vi "OxfordDC_2Channel_ITC503_LKS331_2SRS830.vi"() -> ()   [LabVIEW 2014]
uses:
  <vilib>/Utility/file.llb/Write To Spreadsheet File (DBL).vi
  Lake Shore Cryotronics 370/Lake Shore Cryotronics 370.lvlib
panel:
  out "Probe Temp":dbl format="%.3f"
  out "Cryostat Temp":dbl format="%.3f"
  in  "Tab Control":enum32{"Page 1", "Page 3"}(tab)
  in  "Start T":dbl=130.0
  in  "T Step":dbl=1.0
  in  "End T":dbl
  in  "Mid T":dbl
  in  "T Step 2":dbl=1.0
  in  "Seconds for Stability":dbl=200.0
  in  "SRS830_1\nAddress":i16
  in  "SRS830_2\nAddress":i16
  in  "Save file path":path
  in  "error in (no error)":errorcluster
  out "error out":errorcluster
  in  "Amplitude":dbl=0.75
  in  "Delay Time (s)":dbl=0.4
  in  "Frequency":dbl=0.1
  in  "Offset":dbl=3.0
  in  "Phase":dbl
  in  "Amplifier Offset":dbl=0.1 caption="Frequency"
  in  "Amplifier Gain":dbl=0.1 caption="Frequency"
  in  "Setpoint Proximity":dbl=0.01 format="%#.3g"
  in  "Required Stability":dbl=0.002 format="%#.4g"
  in  "ITC503":refnum<visa-resource-name>
  in  "LKS 370":refnum<visa-resource-name>
  out "XY Graph 3":cluster{dbl, dbl}[](graph) caption="SRS2"
  out "XY Graph 4":cluster{dbl, dbl}[](graph) caption="SRS1"
  out "XY Graph 5":cluster{dbl, dbl}[](graph) caption="LR700"
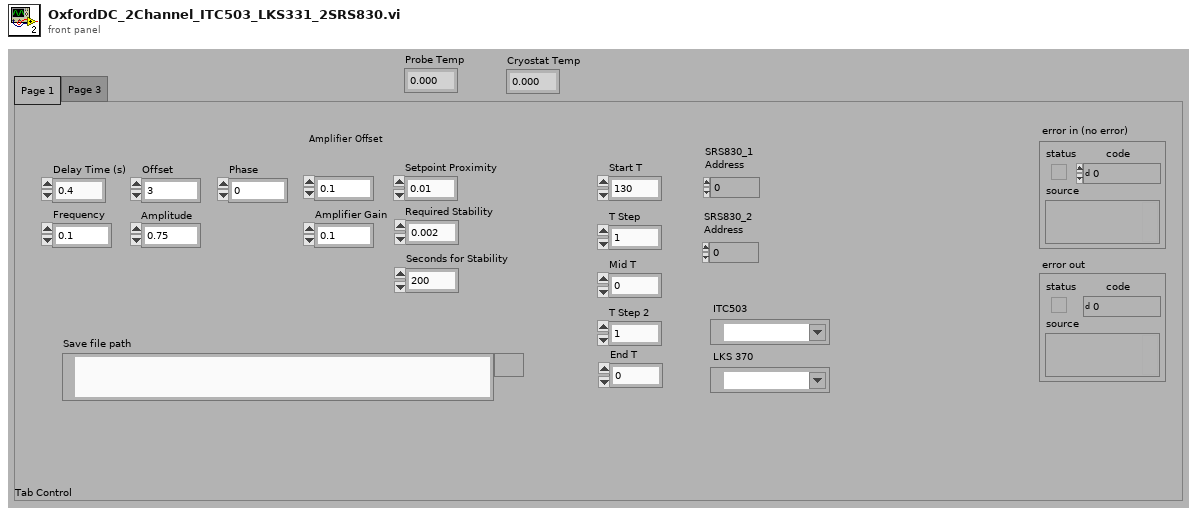
[diagram p1: front panel]
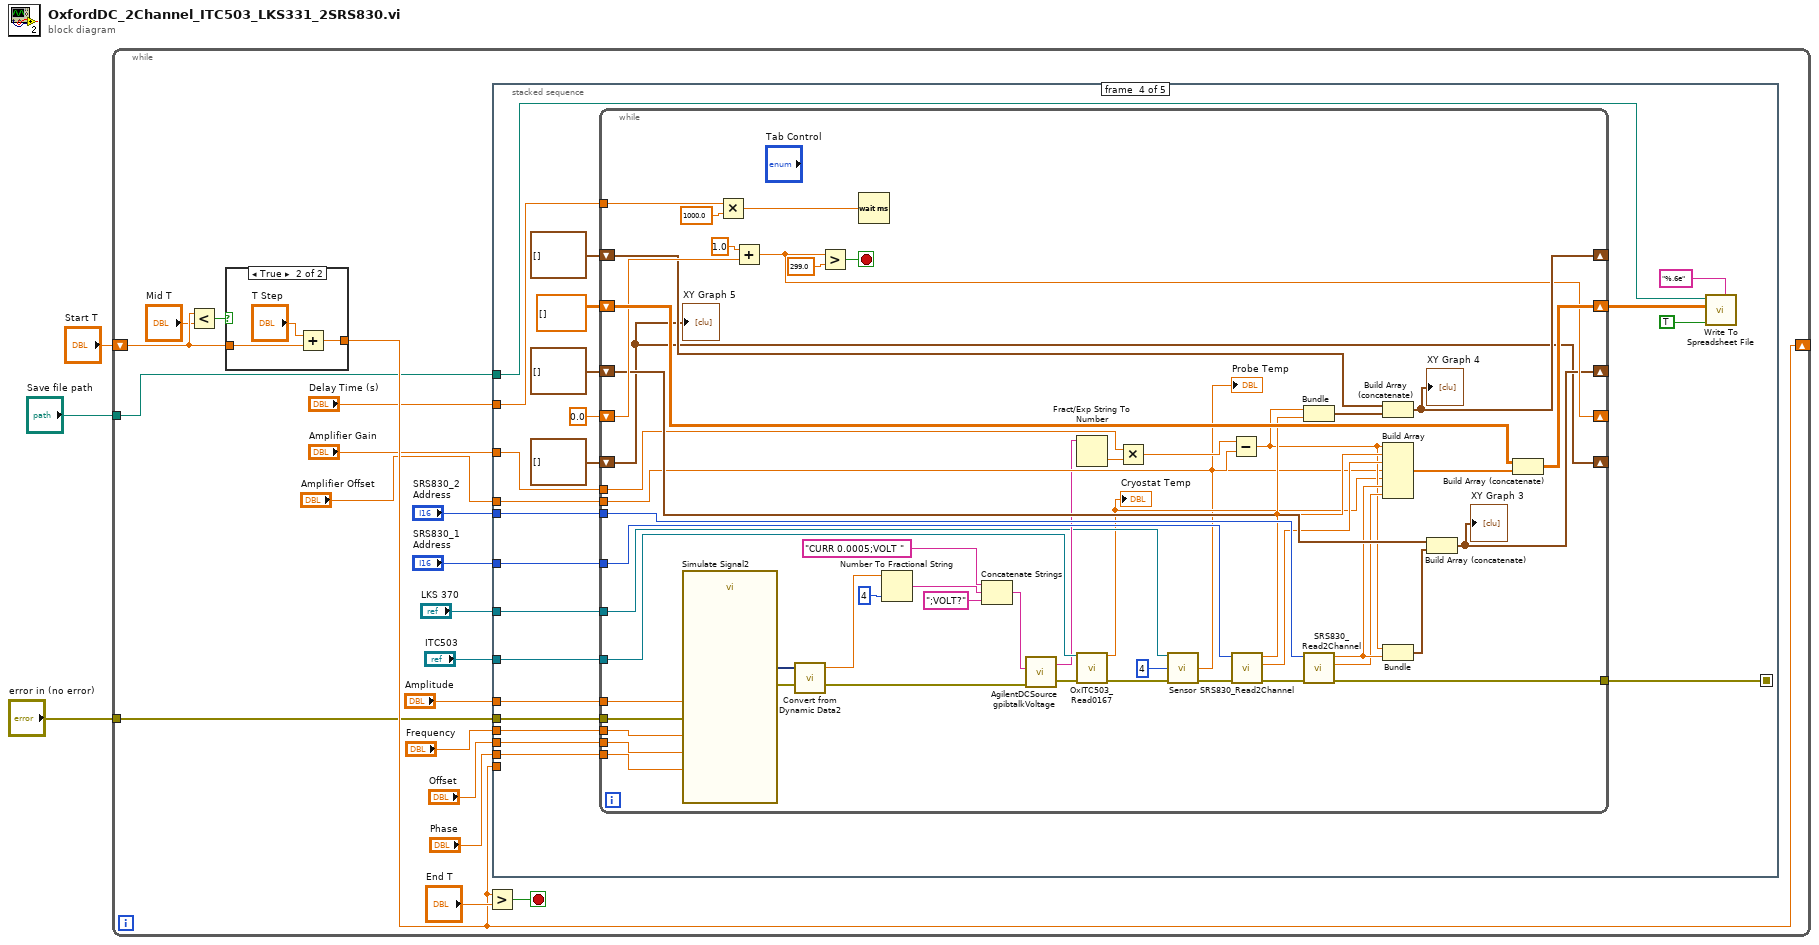
[diagram p0: block diagram]
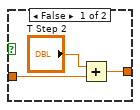
[diagram p2: hidden frame]
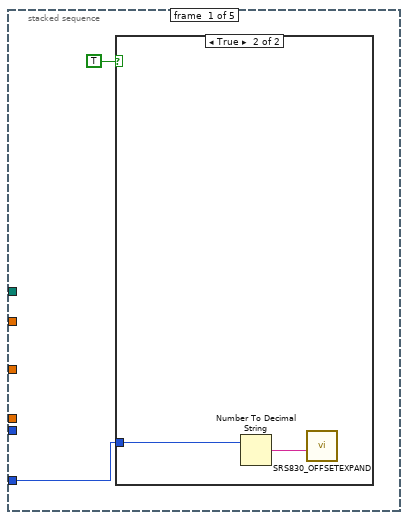
[diagram p3: hidden frame]
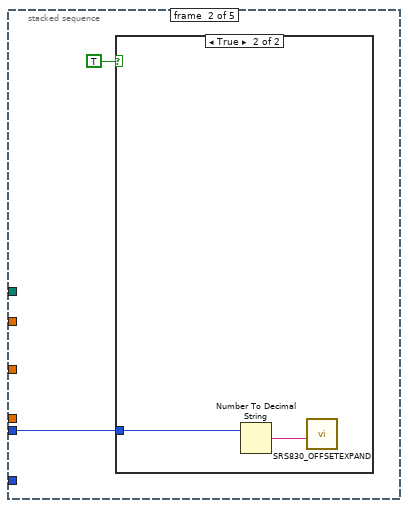
[diagram p5: hidden frame]
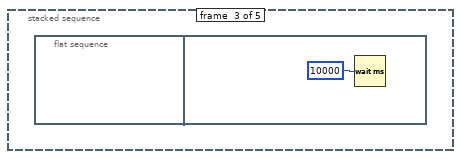
[diagram p7: hidden frame]
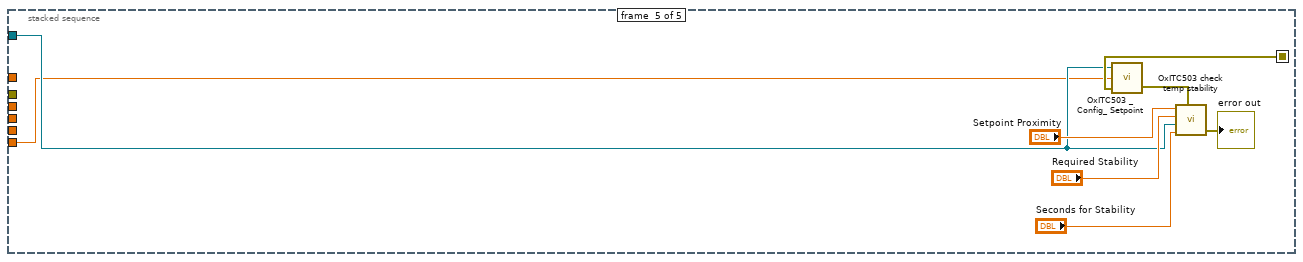
[diagram p8: hidden frame]
diagram:
  n1 = while {
    shift-right: [w17] -> _
    shift-left: "Start T" -> [w20]
    tunnel: "error in (no error)" -> [w16]
    tunnel: "Save file path" -> [w6]
    stop <- w22 stop-if-true
    n2 = Less?(x=w20, y="Mid T") -> (x < y?=w21:bool)
    n3 = case shown="True" w21 {
      tunnel: w20 -> [w24 w27]
      tunnel: [w23 w26] -> w17
      frame False {
        n4 = Add(x="T Step 2", y=w24) -> (x+y=w23:dbl)
      }
      frame True {
        n5 = Add(x="T Step", y=w27) -> (x+y=w26:dbl)
      }
    }
    n6 = Greater?(x=w17, y="End T") -> (0:w22:bool)
    n7 = stacked-sequence {
      seq-local: [_ _ _ w55 _] -> [_ _ _ _ w116]
      tunnel: w17 -> [_ _ _ _ w113]
      tunnel: w16 -> [_ _ _ w56 _]
      tunnel: "SRS830_1\nAddress" -> [w30 _ _ w53 _]
      tunnel: "SRS830_2\nAddress" -> [_ w34 _ w52 _]
      tunnel: "Amplitude" -> [_ _ _ w51 _]
      tunnel: "Frequency" -> [_ _ _ w50 _]
      tunnel: "Offset" -> [_ _ _ w49 _]
      tunnel: "Phase" -> [_ _ _ w48 _]
      tunnel: "Delay Time (s)" -> [_ _ _ w47 _]
      tunnel: "Amplifier Gain" -> [_ _ _ w46 _]
      tunnel: "Amplifier Offset" -> [_ _ _ w45 _]
      tunnel: w6 -> [_ _ _ w41 _]
      tunnel: "LKS 370" -> [_ _ _ w38 _]
      tunnel: "ITC503" -> [_ _ _ w39 w114]
      frame #0 {
        n8 = case shown="True" TRUE {
          tunnel: w30 -> [_ w31]
          frame False {
          }
          frame True {
            n9 = Number To Decimal String(number=w31) -> (decimal integer string=w32:string)  [unwired: 1 in]
            n10 = call "SRS830_OFFSETEXPAND.vi"("address string"=w32) -> ()  [unwired: 11 in]
          }
        }
      }
      frame #1 {
        n11 = case shown="True" TRUE {
          tunnel: w34 -> [_ w35]
          frame False {
          }
          frame True {
            n12 = Number To Decimal String(number=w35) -> (decimal integer string=w36:string)  [unwired: 1 in]
            n13 = call "SRS830_OFFSETEXPAND.vi"("address string"=w36) -> ()  [unwired: 11 in]
          }
        }
      }
      frame #2 {
        n14 = flat-sequence {
          frame #0 {
          }
          frame #1 {
            n15 = Wait (ms)(milliseconds to wait=10000) -> ()  [unwired: 1 out]
          }
        }
      }
      frame #3 {
        n16 = while {
          shift-right: [w105] -> _
          shift-left: cluster{dbl, dbl}[] [] -> [w91]
          shift-right: [w103] -> w42
          shift-left: dbl[][] [] -> [w104]
          shift-right: [w99] -> _
          shift-left: 0.0 -> [w102]
          tunnel: w56 -> [w94]
          tunnel: [w70] -> w55
          shift-right: [w80] -> _
          shift-left: cluster{dbl, dbl}[] [] -> [w89]
          tunnel: w53 -> [w79]
          tunnel: w52 -> [w78]
          tunnel: w51 -> [w87]
          tunnel: w50 -> [w86]
          tunnel: w49 -> [w85]
          tunnel: w48 -> [w84]
          tunnel: w47 -> [w83]
          tunnel: w46 -> [w82]
          tunnel: w45 -> [w73]
          shift-right: [w69] -> _
          shift-left: cluster{dbl, dbl}[] [] -> [w69]
          tunnel: w39 -> [w68]
          tunnel: w38 -> [w62]
          stop <- w100 stop-if-true
          n17 = call "Simulate Signal2"("Offset"=w85, "Frequency"=w86, "Amplitude"=w87, "Phase"=w84, "error in (no error)"=w94) -> ("Triangle"=w112:dynamicdata, "error out"=w93:errorcluster)  [unwired: 9 in]
          n18 = Multiply(x=w83, y=1000.0) -> (x*y=w96:dbl)
          n19 = Add(x=1.0, y=w102) -> (x+y=w99:dbl)
          n20 = call "Convert from Dynamic Data2"("Dynamic Data Type"=w112) -> ("Scalar"=w111:dbl)  [unwired: 3 in]
          n21 = Greater?(x=w99, y=299.0) -> (0:w100:bool)
          n22 = Wait (ms)(milliseconds to wait=w96) -> ()  [unwired: 1 out]
          n23 = Number To Fractional String(number=w111, precision (6)=4) -> (F-format string=w110:string)  [unwired: 2 in]
          n24 = Concatenate Strings("CURR 0.0005;VOLT ", w110, ";VOLT?") -> (w106:string)
          n25 = call "AgilentDCSource gpibtalkVoltage.vi"("error in"=w93, "Send"=w106) -> ("error out"=w63:errorcluster, "read"=w67:string)  [unwired: 2 in]
          n26 = Fract/Exp String To Number(string=w67) -> (number=w88:dbl)  [unwired: 3 in, 1 out]
          n27 = call "OxITC503_Read0167.vi"("VISA session 2"=w68, "error in"=w63) -> ("Temp"=w61:dbl, "error out (no error)"=w64:errorcluster)  [unwired: 8 in, 4 out]
          "Cryostat Temp" <- w61
          n28 = Multiply(x=w82, y=w88) -> (x*y=w95:dbl)
          n29 = call "Sensor.vi"("VISA resource name"=w62, "Channel (1)"=4, "error in (no error)"=w64) -> ("Kelvin Reading"=w60:dbl, "error out"=w65:errorcluster)  [unwired: 8 in, 3 out]
          "Probe Temp" <- w60
          n30 = Subtract(x=w95, y=w73) -> (x-y=w71:dbl)
          n31 = call "SRS830_Read2Channel.vi"("error in (no error)"=w65, "Lock in\nGPIB Address"=w79) -> ("error out"=w77:errorcluster, "Ch_OUTP3"=w72:dbl, "Ch_OUTR1"=w74:dbl)  [unwired: 7 in]
          n32 = Bundle(w71, "Ch_OUTR1"=w74) -> (w90:cluster{dbl, "Ch_OUTR1":dbl})  [unwired: 1 in]
          n33 = call "SRS830_Read2Channel.vi"("error in (no error)"=w77, "Lock in\nGPIB Address"=w78) -> ("error out"=w70:errorcluster, "Ch_OUTP3"=w75:dbl, "Ch_OUTR1"=w76:dbl)  [unwired: 7 in]
          n34 = Build Array (concatenate)(w91, w90) -> (w105:cluster{dbl, "Ch_OUTR1":dbl}[])
          "XY Graph 4" <- w105
          n35 = Build Array(w71, w74, w72, w60, w61, w76, w75) -> (w81:dbl[])
          n36 = Bundle(w71, "Ch_OUTR1"=w76) -> (w92:cluster{dbl, "Ch_OUTR1":dbl})  [unwired: 1 in]
          n37 = Build Array (concatenate)(w89, w92) -> (w80:cluster{dbl, "Ch_OUTR1":dbl}[])
          "XY Graph 3" <- w80
          n38 = Build Array (concatenate)(w104, w81) -> (w103:dbl[][])
          "XY Graph 5" <- w69
        }
        n39 = call-poly <vilib>:"Write To Spreadsheet File.vi"("format (%.3f)"="%.6e", "append to file? (new file:F)"=TRUE, "2D data"=w42, "file path (dialog if empty)"=w41) -> ()  [unwired: 4 in, 1 out]
      }
      frame #4 {
        n40 = call "OxITC503 _Config_ Setpoint.vi"("error in"=w116, "Setpoint"=w113, "VISA session"=w114) -> ("error out (no error)"=w115:errorcluster)  [unwired: 1 out]
        n41 = call "OxITC503 check temp stability.vi"("Set point proximity"="Setpoint Proximity", "Stability"="Required Stability", "OxfordITC503s"=w114, "seconds to wait"="Seconds for Stability", "error in"=w115) -> ("error out"=→"error out":errorcluster)  [unwired: 2 in]
      }
    }
  }
